vi "SPI Slave Write Bytes.vi"(6 "TimeOutMs":i32, 7 "WriteLen":i32, 9 "pWriteData":u8, 10 "SPIIndex":i32, 11 "DevHandle":i32) -> (1 "pWriteData out":u8, 3 "function return":i32)   [LabVIEW 2010, in "usb2spi.lvlib"]
doc: "int WINAPI SPI_SlaveWriteBytes(int DevHandle,int SPIIndex,unsigned char *pWriteData,int WriteLen,int TimeOutMs);"
uses:
  usb2spi.lvlib
  USB2XXX.dll
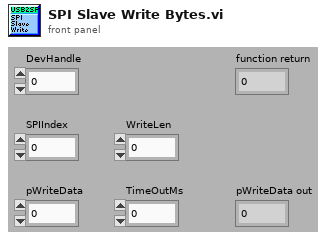
[diagram p1: front panel]
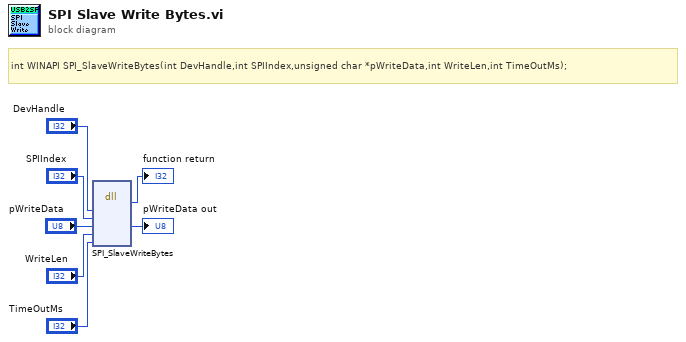
[diagram p0: block diagram]
diagram:
  # "int WINAPI SPI_SlaveWriteBytes(int DevHandle,int SPIIndex,unsigned char *pWriteData,int WriteLen,int TimeOutMs);"
  n1 = dll-call lib="G:/OtherWork/USB2XXX_Example/trunk/Labview/PublicFiles/usb2spi/USB2XXX.*" fn="SPI_SlaveWriteBytes"("DevHandle"="DevHandle", "SPIIndex"="SPIIndex", "pWriteData"="pWriteData", "WriteLen"="WriteLen", "TimeOutMs"="TimeOutMs") -> (→"function return":i32, "pWriteData"=→"pWriteData out":u8)  [unwired: 7 in, 2 out]
